vi "set array to zero.vi"   [LabVIEW 2012, in "common.lvlib"]
uses:
  common.lvlib
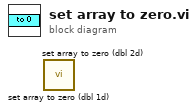
[diagram p0: block diagram]
diagram:
  n1 = call "set array to zero (dbl 1d).vi"() -> ()  [unwired: 1 in, 1 out]
  n2 = call "set array to zero (dbl 2d).vi"() -> ()  [unwired: 1 in, 1 out]
